vi "Inhibit Bus A.vi"(5 "Component ID":u8, 7 "FPGA Interface":refnum<class "FPGA Interface.lvclass">, 8 "error in (no error)":errorcluster, 10 "Inhibit Bus A?":bool, 11 "Remote Terminal in":refnum<class "Remote Terminal.lvclass">) -> (0 "error out":errorcluster, 3 "Remote Terminal out":refnum<class "Remote Terminal.lvclass">)   [LabVIEW 2020, in "BCI-1553 API.lvlib" / "Remote Terminal.lvclass"]
doc: "Inhibits or enables the operation of Bus A for this Remote Terminal."
uses:
  Remote Terminal.lvclass
  Dependencies/FPGA Interface/FPGA Interface.lvclass
  Remote Terminal.lvclass/Remote Terminal.ctl
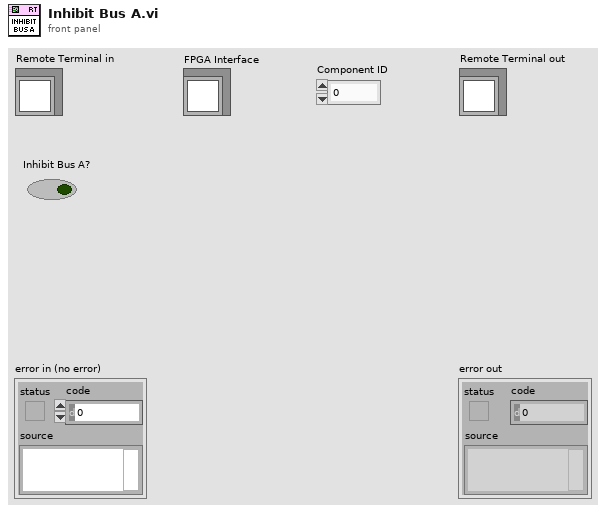
[diagram p1: front panel]
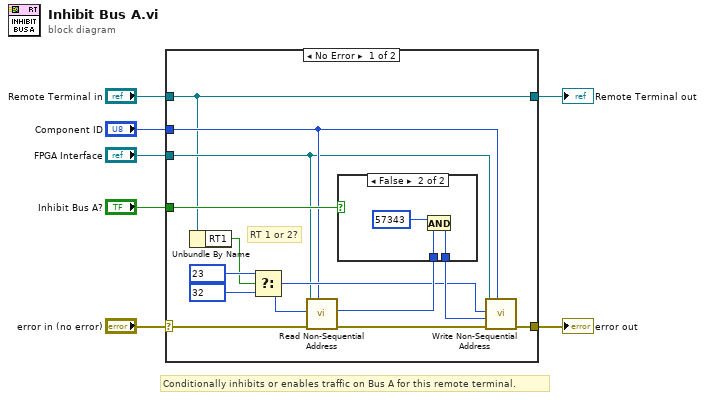
[diagram p0: block diagram]
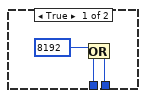
[diagram p2: hidden frame]
diagram:
  # "Conditionally inhibits or enables traffic on Bus A for this remote terminal."
  n1 = case shown="No Error" "error in (no error)" {
    selector: "error in (no error)" -> [w17 w28]
    tunnel: [w16 w28] -> w1
    tunnel: "Remote Terminal in" -> [w9 w27]
    tunnel: [w9 w27] -> w7
    tunnel: "Component ID" -> [w11 _]
    tunnel: "FPGA Interface" -> [w10 _]
    tunnel: "Inhibit Bus A?" -> [w12 _]
    frame No Error {
      # "RT 1 or 2?"
      n2 = Unbundle By Name(w9) -> ("RT1"=w8:bool)
      n3 = Select(t=u16 23 ("Address"), s=w8, f=u16 32 ("Address")) -> (s? t:f=w13:u16)
      n4 = call-dynamic "Read Non-Sequential Address.vi"("Target IC (1-8)"=w11, "error in (no error)"=w17, "Address"=w13, "FPGA Interface in"=w10) -> ("error out"=w18:errorcluster, "Data"=w19:u16)  [unwired: 6 in]
      n5 = case shown="False" w12 {
        tunnel: [w23 w26] -> w20
        tunnel: w19 -> [w22 w25]
        frame True {
          n6 = Or(x=u16 8192 ("Address"), y=w22) -> (x .or. y?=w23:u16)
        }
        frame False {
          n7 = And(x=u16 57343 ("Address"), y=w25) -> (x .and. y?=w26:u16)
        }
      }
      n8 = call-dynamic "Write Non-Sequential Address.vi"("Target IC (1-8)"=w11, "error in (no error)"=w18, "Data"=w20, "Address"=w13, "FPGA Interface in"=w10) -> ("error out"=w16:errorcluster)  [unwired: 6 in]
    }
    frame Error {
    }
  }
  "error out" <- w1
  "Remote Terminal out" <- w7
